vi "updateM300NTCENTwithMESEquip.vi"() -> ()   [LabVIEW 2012]
uses:
  <vilib>/addons/database/Connection.llb/DB Tools Open Connec (Path).vi
  <vilib>/addons/database/Connection.llb/Conn Execute.vi
  <vilib>/addons/database/Recordset.llb/Rec Fetch Recordset Data (R).vi
  <vilib>/addons/database/Recordset.llb/Rec Destroy - Connection.vi
  <vilib>/addons/database/_DB Variant To Data/Database Variant To Data.xnode
  <vilib>/addons/database/NI_Database_API.lvlib
panel:
  out "error out":errorcluster
  out "concatenated string":string
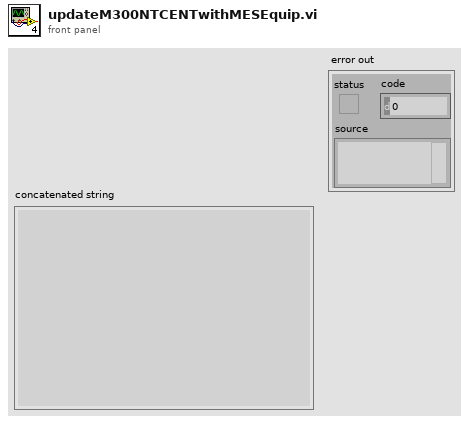
[diagram p1: front panel]
types:
  T1 = typedef "NI_Database_API.lvlib/Conn ObjectReference.ctl" = refnum<k1>
  T2 = typedef "NI_Database_API.lvlib/Rec ObjectReference.ctl" = refnum<k1>
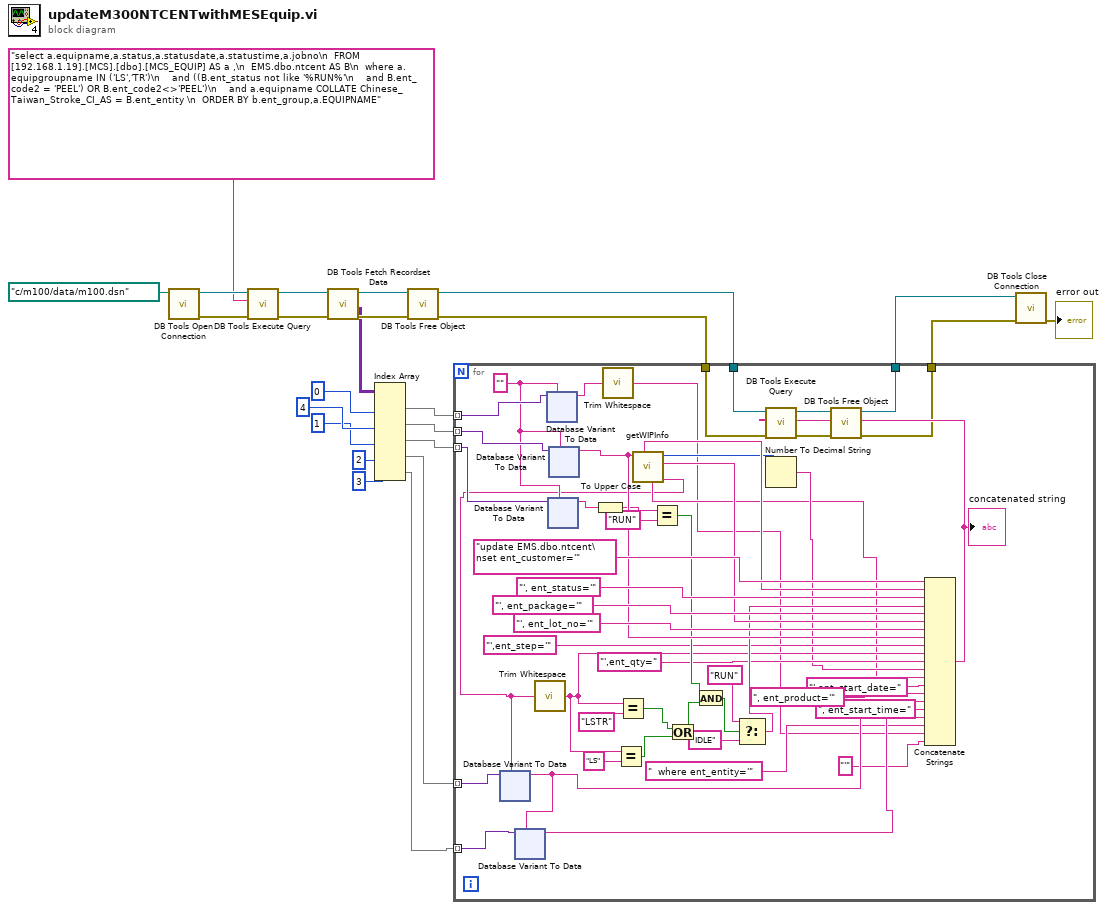
[diagram p0: block diagram]
diagram:
  n1 = call-poly <vilib>:"DB Tools Open Connection.vi"("connection information"=path "c:/m100/data/m100.dsn") -> ("error out"=w24:errorcluster, "connection reference"=w23:T1)  [unwired: 7 in]
  n2 = call-poly <vilib>:"DB Tools Execute Query.vi"("error in (no error)"=w24, "SQL query"="select a.equipname,a.status,a.statusdate,a.statustime,a.jobno\n  FROM [192.168.1.19].[MCS].[dbo].[MCS_EQUIP] AS a ,\n  EMS.dbo.ntcent AS B\n  where a.equipgroupname IN ('LS','TR')\n    and ((B.ent_status not like '%RUN%'\n    and B.ent_code2 = 'PEEL') OR B.ent_code2<>'PEEL')\n    and a.equipname COLLATE Chinese_Taiwan_Stroke_CI_AS = B.ent_entity \n  ORDER BY b.ent_group,a.EQUIPNAME", "connection reference"=w23) -> ("error out"=w20:errorcluster, "recordset reference"=w22:T2)  [unwired: 5 in]
  n3 = call-poly <vilib>:"DB Tools Fetch Recordset Data.vi"("error in (no error)"=w20, "recordset reference"=w22) -> ("error out"=w19:errorcluster, "recordset data"=w16:variant[][], "recordset reference out"=w21:T2)  [unwired: 3 in]
  n4 = Index Array(array=w16, index (col) #1=0 ("disabled index (col)"), index (col) #2=4 ("index (col)"), index (col) #3=1 ("index (col)"), index (col) #4=2 ("index (col)"), index (col) #5=3 ("index (col)")) -> (element #1=w12:variant[], element #2=w11:variant[], element #3=w10:variant[], element #4=w2:variant[], element #5=w1:variant[])  [unwired: 5 in]
  n5 = call-poly <vilib>:"DB Tools Free Object.vi"("error in (no error)"=w19, "recordset reference"=w21) -> ("error out"=w8:errorcluster, "connection reference"=w9:T1)  [unwired: 8 in]
  n6 = for {
    tunnel: w12 -> [w73] mode=indexing
    tunnel: w11 -> [w72] mode=indexing
    tunnel: w10 -> [w71] mode=indexing
    tunnel: w9 -> [w62]
    tunnel: w8 -> [w61]
    tunnel: [w58] -> w7
    tunnel: [w57] -> w6
    tunnel: w2 -> [w33] mode=indexing
    tunnel: w1 -> [w30] mode=indexing
    w70 = ""
    n7 = xnode "Database Variant To Data"("database variant"=w73, "type"=w70) -> ("data"=w56:string)  [unwired: 1 in, 1 out]
    n8 = xnode "Database Variant To Data"("database variant"=w71, "type"=w70) -> ("data"=w54:string)  [unwired: 1 in, 1 out]
    n9 = xnode "Database Variant To Data"("database variant"=w72, "type"=w70) -> ("data"=w55:string)  [unwired: 1 in, 1 out]
    n10 = To Upper Case(1:w54) -> (0:w49:string)
    n11 = call <vilib>:"Trim Whitespace.vi"("string"=w56) -> ("trimmed string"=w26:string)  [unwired: 1 in]
    n12 = call "getWIPInfo.vi"("Lotno"=w55) -> ("step"=w32:string, "Package"=w65:string, "data"=w38:i32, "Product"=w35:string, "CustomerID"=w68:string)  [unwired: 4 in, 2 out]
    n13 = xnode "Database Variant To Data"("database variant"=w33, "type"=w32) -> ("data"=w29:string)  [unwired: 1 in, 1 out]
    n14 = xnode "Database Variant To Data"("database variant"=w30, "type"=w29) -> ("data"=w28:string)  [unwired: 1 in, 1 out]
    n15 = call <vilib>:"Trim Whitespace.vi"("string"=w32) -> ("trimmed string"=w40:string)  [unwired: 1 in]
    n16 = Equal?(x=w40, y="LS") -> (x = y?=w50:bool)
    n17 = Equal?(x=w40, y="LSTR" ("regular expression")) -> (x = y?=w51:bool)
    n18 = Equal?(x=w49, y="RUN") -> (x = y?=w47:bool)
    n19 = Or(x=w51, y=w50) -> (x .or. y?=w46:bool)
    n20 = And(x=w47, y=w46) -> (x .and. y?=w45:bool)
    n21 = Select(t="RUN", s=w45, f="IDLE") -> (s? t:f=w42:string)
    n22 = Number To Decimal String(number=w38) -> (decimal integer string=w37:string)  [unwired: 1 in]
    n23 = Concatenate Strings("update EMS.dbo.ntcent\nset ent_customer='" ("string"), w68, "', ent_status='" ("string"), w42, "', ent_package='" ("string"), w65, "', ent_lot_no='" ("string"), w55, "',ent_step='" ("string"), w40, "',ent_qty=" ("string"), w37, ", ent_product='" ("string"), w35, "',ent_start_date=" ("string"), w29, ", ent_start_time=" ("string"), w28, "  where ent_entity='" ("string"), w26, "'" ("string")) -> (w63:string)
    "concatenated string" <- w63
    n24 = call-poly <vilib>:"DB Tools Execute Query.vi"("error in (no error)"=w61, "SQL query"=w63, "connection reference"=w62) -> ("error out"=w59:errorcluster, "recordset reference"=w60:T2)  [unwired: 5 in]
    n25 = call-poly <vilib>:"DB Tools Free Object.vi"("error in (no error)"=w59, "recordset reference"=w60) -> ("error out"=w57:errorcluster, "connection reference"=w58:T1)  [unwired: 8 in]
  }
  n26 = call <vilib>:"DB Tools Close Connection.vi"("error in (no error)"=w6, "connection reference"=w7) -> ("error out"=→"error out":errorcluster)  [unwired: 5 in]
